vi "PWM FPGA Dephasing_control loop.vi"() -> ()   [LabVIEW 2013]
uses:
  <vilib>/eio/EIONode/EIONode.xnode
  <vilib>/rvi/eio/common/nirviEmuTemplateMethod_errors.vi
panel:
  in  "Tab Control":enum32{"Page 1", "Page 2"}(tab)
  in  "Control":T1={"Pulse Lenght DIO3"=10000, "Pulse Period 3"=20000, "Dephasing 3"=0, "Pulse Lenght DIO0"=10000, "Pulse Period 0"=20000, "Dephasing 0"=0}
  in  "Update":bool
  out "Cluster":T1
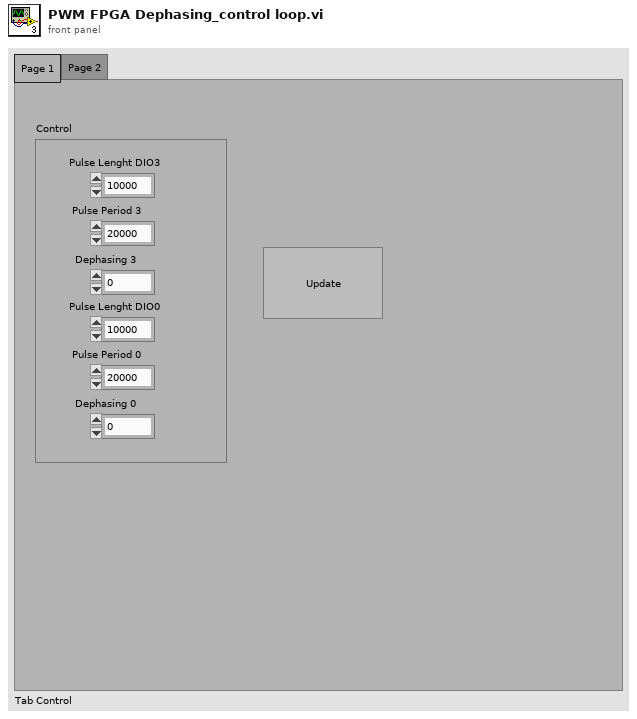
[diagram p1: front panel]
types:
  T1 = cluster{"Pulse Lenght DIO3":i16, "Pulse Period 3":i16, "Dephasing 3":i16, "Pulse Lenght DIO0":i16, "Pulse Period 0":i16, "Dephasing 0":i16}
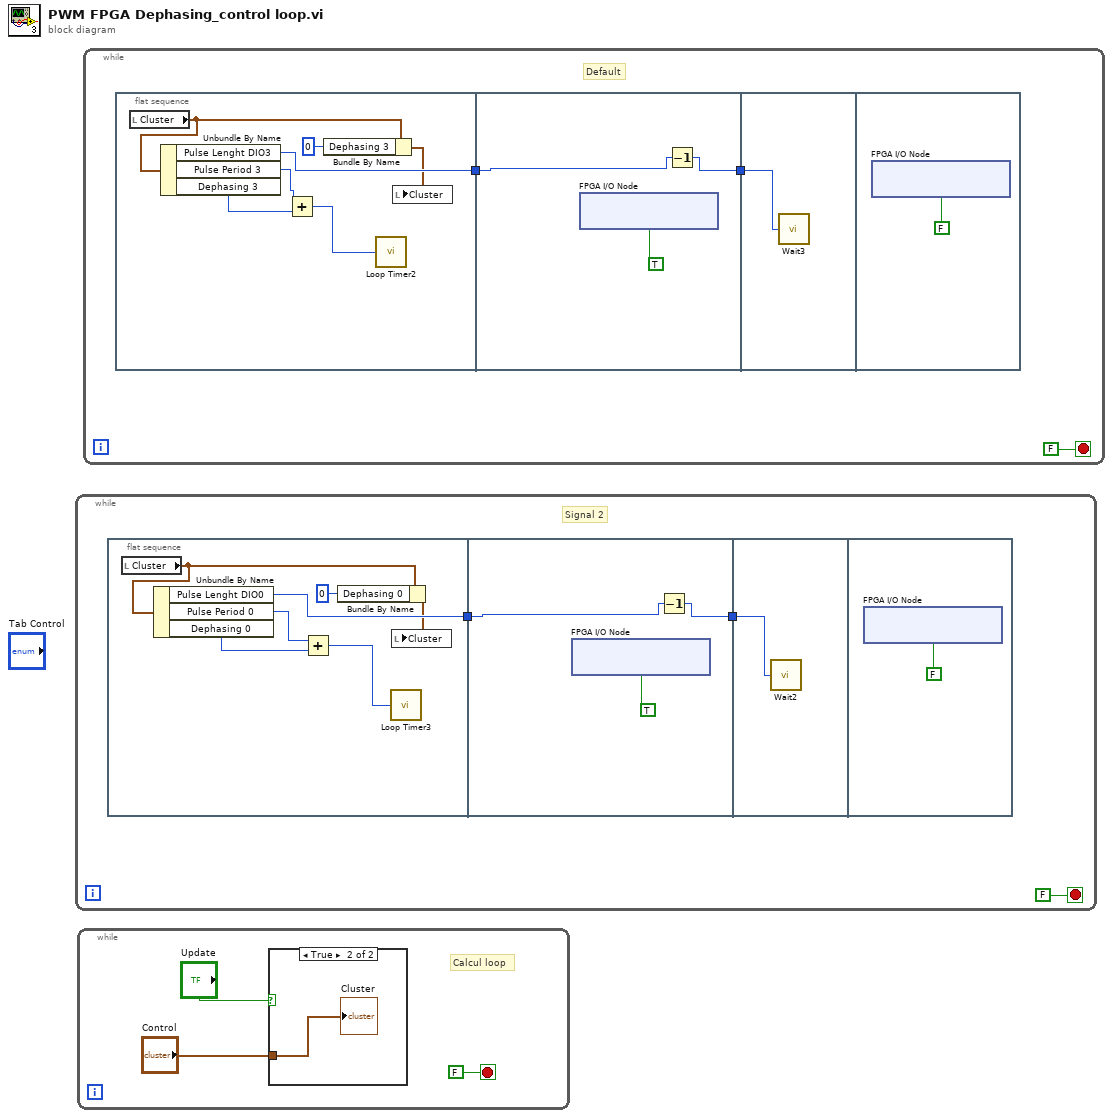
[diagram p0: block diagram]
diagram:
  n1 = while {
    stop <- FALSE stop-if-true
    # "Signal 2"
    n2 = flat-sequence {
      tunnel: [w10] -> w2
      tunnel: w2 -> [w11]
      tunnel: [w12] -> w1
      tunnel: w1 -> [w14]
      frame #0 {
        n3 = local read "Cluster"() -> (w9:T1)
        n4 = Unbundle By Name(w9) -> ("Pulse Lenght DIO0"=w10:i16, "Pulse Period 0"=w6:i16, "Dephasing 0"=w5:i16)
        n5 = Add(x=w6, y=w5) -> (x+y=w4:i16)
        n6 = Bundle By Name(cluster=w9, "Dephasing 0"=i16 0 ("Dephasing 3")) -> (w7:T1)
        n7 = call "Loop Timer3"("Count(Ticks)"=w4) -> ()  [unwired: 1 out]
        n8 = local write "Cluster"(w7) -> ()
      }
      frame #1 {
        n9 = xnode "FPGA I/O Node"("ConnectorC/DIO0"=TRUE ("ConnectorC/DIO7")) -> ()  [unwired: 1 in, 1 out]
        n10 = Decrement(x=w11) -> (x-1=w12:i16)
      }
      frame #2 {
        n11 = call "Wait2"("Count(Ticks)"=w14) -> ()  [unwired: 1 out]
      }
      frame #3 {
        n12 = xnode "FPGA I/O Node"("ConnectorC/DIO0"=FALSE ("ConnectorC/DIO7")) -> ()  [unwired: 1 in, 1 out]
      }
    }
  }
  n13 = while {
    stop <- FALSE stop-if-true
    # "Calcul loop"
    n14 = case shown="True" "Update" {
      tunnel: "Control" -> [_ w19]
      frame False {
      }
      frame True {
        "Cluster" <- w19
      }
    }
  }
  n15 = while {
    stop <- FALSE stop-if-true
    # "Default"
    n16 = flat-sequence {
      tunnel: [w29] -> w21
      tunnel: w21 -> [w30]
      tunnel: [w31] -> w20
      tunnel: w20 -> [w33]
      frame #0 {
        n17 = local read "Cluster"() -> (w23:T1)
        n18 = Unbundle By Name(w23) -> ("Pulse Lenght DIO3"=w29:i16, "Pulse Period 3"=w27:i16, "Dephasing 3"=w28:i16)
        n19 = Add(x=w27, y=w28) -> (x+y=w26:i16)
        n20 = Bundle By Name(cluster=w23, "Dephasing 3"=i16 0) -> (w24:T1)
        n21 = call "Loop Timer2"("Count(Ticks)"=w26) -> ()  [unwired: 1 out]
        n22 = local write "Cluster"(w24) -> ()
      }
      frame #1 {
        n23 = xnode "FPGA I/O Node"("ConnectorC/DIO3"=TRUE ("ConnectorC/DIO7")) -> ()  [unwired: 1 in, 1 out]
        n24 = Decrement(x=w30) -> (x-1=w31:i16)
      }
      frame #2 {
        n25 = call "Wait3"("Count(Ticks)"=w33) -> ()  [unwired: 1 out]
      }
      frame #3 {
        n26 = xnode "FPGA I/O Node"("ConnectorC/DIO3"=FALSE ("ConnectorC/DIO7")) -> ()  [unwired: 1 in, 1 out]
      }
    }
  }
